vi "Write FolderName.vi"(8 "error in (no error)":errorcluster, 10 "FolderName":path, 11 "Folder_Mgmt in":refnum<class "Folder_Mgmt.lvclass">) -> (0 "error out":errorcluster, 3 "Folder_Mgmt out":refnum<class "Folder_Mgmt.lvclass">)   [LabVIEW 2016, in "Folder_Mgmt.lvclass"]
uses:
  Folder_Mgmt.lvclass
  Folder_Mgmt.lvclass/Folder_Mgmt.ctl
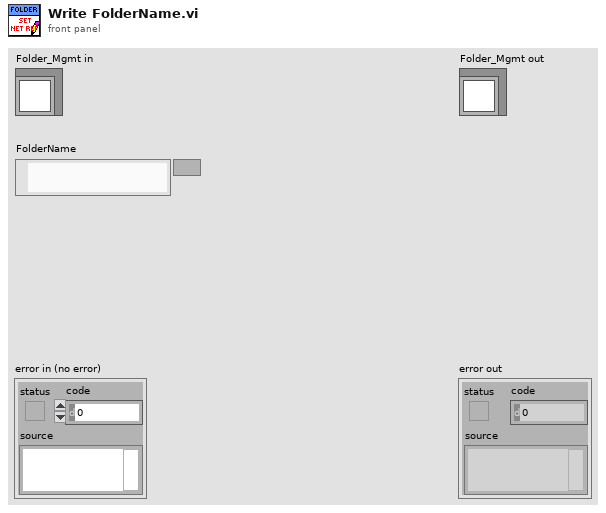
[diagram p1: front panel]
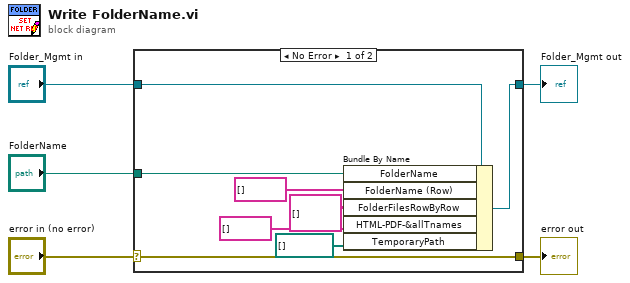
[diagram p0: block diagram]
diagram:
  n1 = case shown="No Error" "error in (no error)" {
    selector: "error in (no error)" -> [w13 w14]
    tunnel: [w13 w14] -> w4
    tunnel: [w11 w15] -> w2
    tunnel: "Folder_Mgmt in" -> [w12 w15]
    tunnel: "FolderName" -> [w10 _]
    frame No Error {
      n2 = Bundle By Name(cluster=w12, "FolderName"=w10, "FolderName (Row)"=string[] [], "FolderFilesRowByRow"=string[][] [], "HTML-PDF-&allTnames"=string[] [], "TemporaryPath"=path[] []) -> (w11:refnum<class "Folder_Mgmt.lvclass">)
    }
    frame Error {
    }
  }
  "error out" <- w4
  "Folder_Mgmt out" <- w2
